vi "Write speeds.vi"(8 "error in (no error)":errorcluster, 10 "speeds":dbl[](array[numeric]), 11 "DelayLine in":refnum<class "DelayLine.lvclass">) -> (0 "error out":errorcluster, 3 "DelayLine out":refnum<class "DelayLine.lvclass">)   [LabVIEW 2020, in "DelayLine.lvclass"]
uses:
  DelayLine.lvclass
  DelayLine.lvclass/DelayLine.ctl
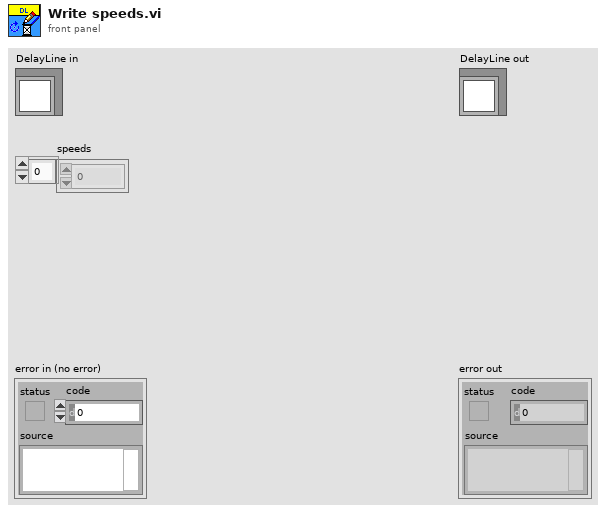
[diagram p1: front panel]
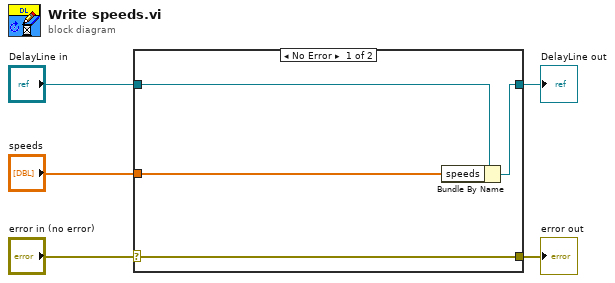
[diagram p0: block diagram]
diagram:
  n1 = case shown="No Error" "error in (no error)" {
    selector: "error in (no error)" -> [w9 w10]
    tunnel: [w9 w10] -> w4
    tunnel: [w7 w11] -> w2
    tunnel: "DelayLine in" -> [w8 w11]
    tunnel: "speeds" -> [w6 _]
    frame No Error {
      n2 = Bundle By Name(cluster=w8, "speeds"=w6) -> (w7:refnum<class "DelayLine.lvclass">)
    }
    frame Error {
    }
  }
  "error out" <- w4
  "DelayLine out" <- w2
